vi "FFT_polynomial_bkg.vi"(8 "Y-column names":string[](array[string])=["col0"], 10 "column extension":string[](array[string])=["summer school 206.006.text"], 11 "Graph array":cluster{"output":dbl[], "output":dbl[]}[](array[cluster])=[{"output"=array[1000 elements], "output"=array[1000 elements]}]) -> ()   [LabVIEW 2025]
uses:
  <vilib>/Analysis/1siggen.llb/Ramp Pattern by Samples.vi
  <vilib>/Analysis/4window.llb/Welch Window (DBL).vi
  <vilib>/Analysis/4window.llb/Triangle Window (DBL).vi
  <vilib>/Analysis/4window.llb/Modified Bartlett-Hanning Window (DBL).vi
  <vilib>/Analysis/4window.llb/Hanning Window (DBL).vi
  <vilib>/Analysis/4window.llb/Hamming Window (DBL).vi
  <vilib>/Analysis/4window.llb/Blackman Window (DBL).vi
  <vilib>/Analysis/2dsp.llb/Power Spectrum (DBL).vi
  <vilib>/Analysis/4window.llb/AllCosWindow (DBL).vi
  <vilib>/Analysis/NI_AALPro.lvlib
  <vilib>/Analysis/NI_AALBase.lvlib
  <vilib>/gmath/NI_Gmath.lvlib
panel:
  in  "length":i32=1000
  in  "index":i32
  in  "bkg removal":enum16{"divide", "subtract"}(ring)
  in  "data":enum16{"spectrum", "1/B plot"}(ring)
  out "1/(x-scale range)":dbl
  in  "show accumulative spectrums":bool
  out "x-array":dbl[](array[numeric])
  in  "export":T1(ring)=enum."write to clipboard"
  in  "data offset":dbl format="%.2e"
  in  "use 1/B for fit":bool
  in  "Bbkg final":dbl=22.0 format="%.2f"
  in  "Bbkg init":dbl=13.0 format="%.2f"
  in  "bkg removal method":enum16{"polynomial", "Cheby poly"}(ring)
  out "raw data/bkg":T2(graph)
  out "FFT spectrum":cluster{"all rows":dbl[], "all rows":dbl[]}[](graph)
  in  "interpol. method":i32(ring)=2 items=["nearest", "linear", "spline", "cubic Hermite", "Lagrange"]
  in  "window":T3(ring)=enum."Hanning"
  in  "stop":bool
  in  "use variables":bool
  in  "Interpolation #":i32=5000
  in  "export results":bool
  out "Field, Freq., Amp":string="0.000E+0\t2.237E+2\r\n"
  out "FFT freq":cluster{"array type (2D Dbl)":dbl[], dbl[]}(graph)={"array type (2D Dbl)"=[0.0], [223.74319564521292]}
  out "FFT amp":cluster{"array type (2D Dbl)":dbl[], dbl[]}(graph)={"array type (2D Dbl)"=[0.0], [8.187351253588833e-05]}
  out "Windowed Signal":cluster{"all rows":dbl[], "all rows":dbl[]}[](graph)
  in  "bkg poly. order":i32=2
  in  "B final":dbl=22.0 format="%.2f"
  in  "B init":dbl=13.0 format="%.2f"
  out "1/B plot after bkg removed":cluster{"all rows":dbl[], "all rows":dbl[]}[](graph)
  in  "variable":string="4.2\n3.5\n3"
  # "Turn on the Show Context Help option ON for\na brief explanation of the controls and graphs."
  # "1. Background removal is done by fitting (normal or Chebyshev polynomial) \n   i) Fitting is done for the range given by 'Bbkg init' and 'Bbkg final'.\n   ii) Background curve is extended to the range give by 'B init' and 'B final'.\n\n2. FFT is done in the range given by 'B init' and 'B final'."
  # "The position and amplitude of the peak will appear on the right two panels. \nOne can zoom in or out to focus on specific peaks."
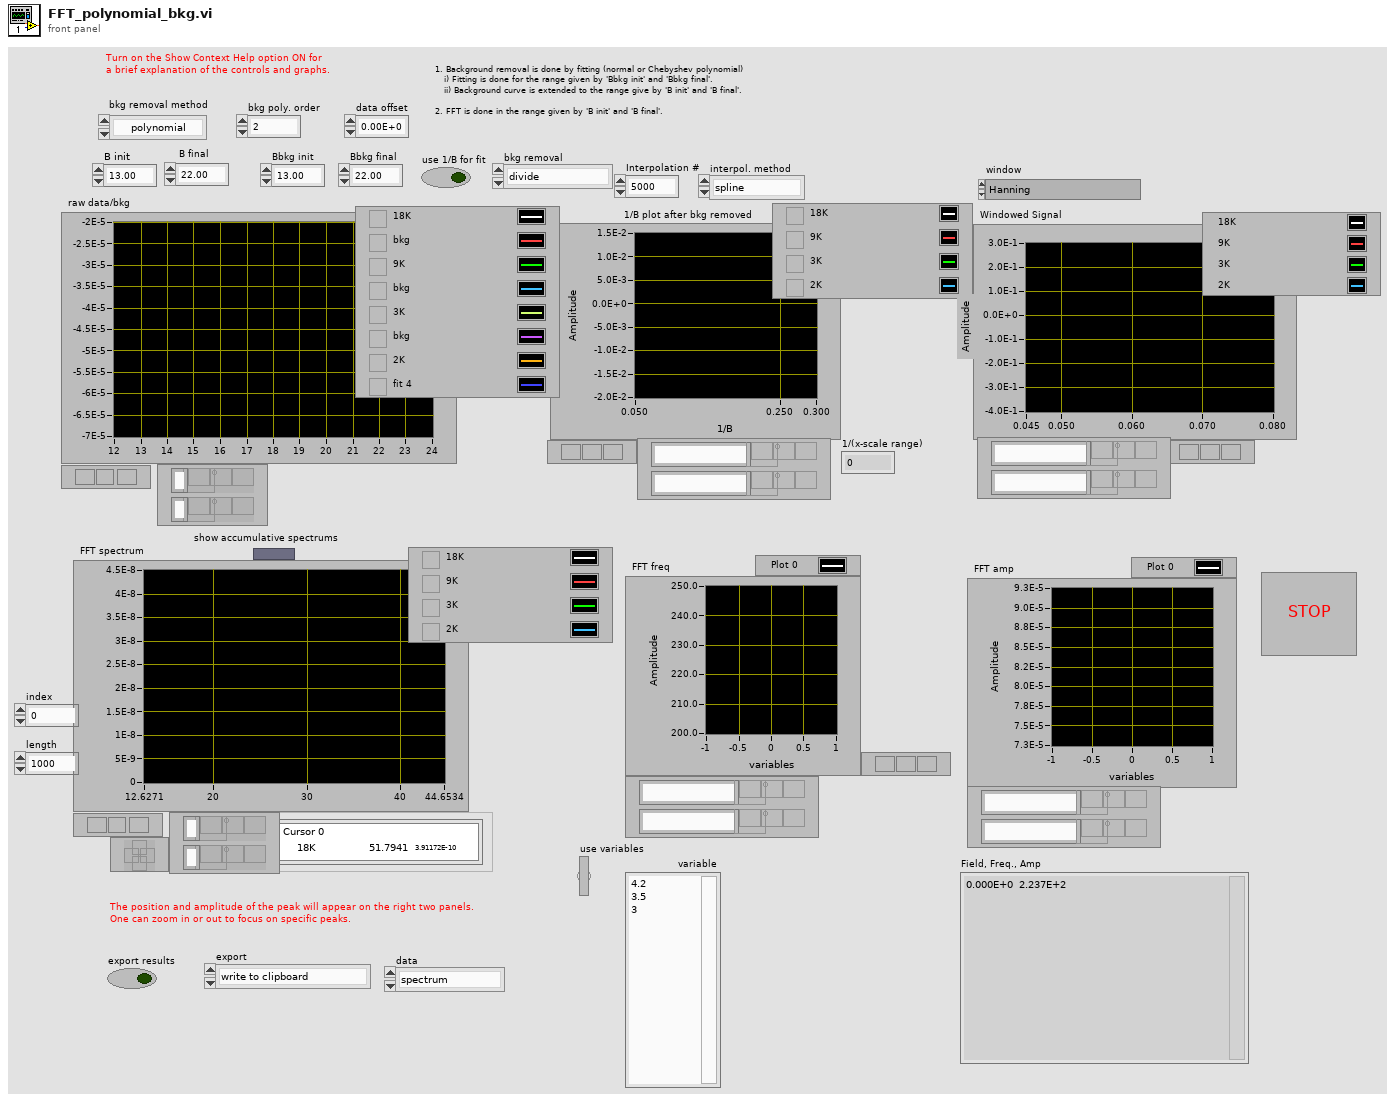
[diagram p1: front panel]
types:
  T1 = enum16{"Save as Ascill file", "write to clipboard", "write to Igor ITX file"}
  T2 = cluster{"Ramp Pattern":dbl[], "Power Spectrum":dbl[]}[]
  T3 = enum16{"none", "Welch", "Triangular", "Bartlett", "Hanning", "Hamming", "Blackmann"}
  T4 = enum16{"Save as Ascill file", "write to clipboard", "do not export"}
  T5 = cluster{"extended B":dbl[], "extended data":dbl[]}
  T6 = cluster{"xi used":dbl[], "Zero Padded Array":dbl[]}
  T7 = cluster{"xi used":dbl[], "Zero Padded Array":dbl[]}[]
  T8 = cluster{"extended B":dbl[], "extended data":dbl[]}[]
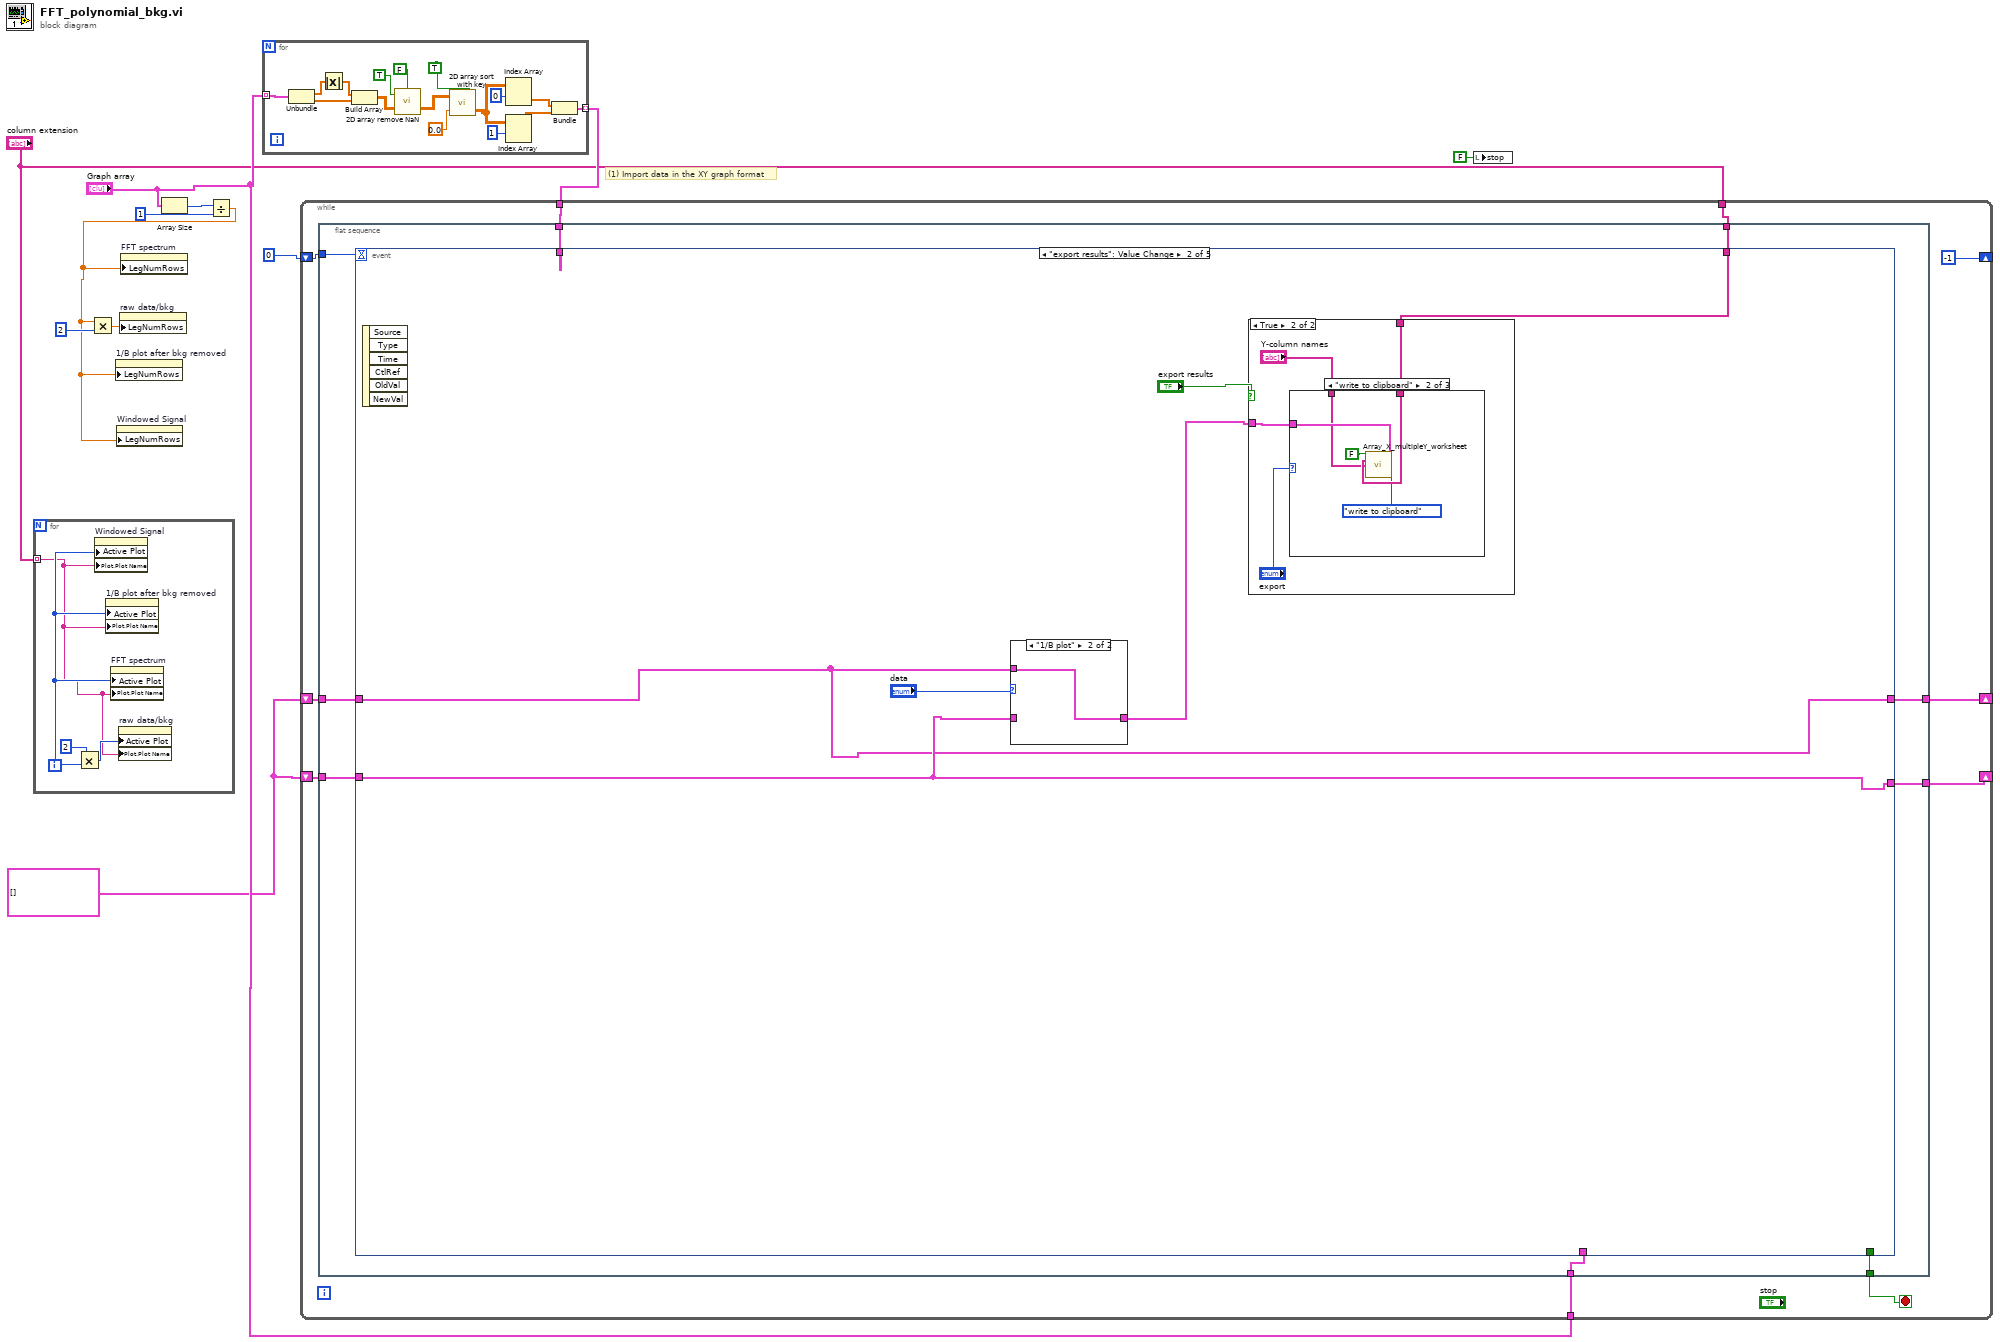
[diagram p0: block diagram]
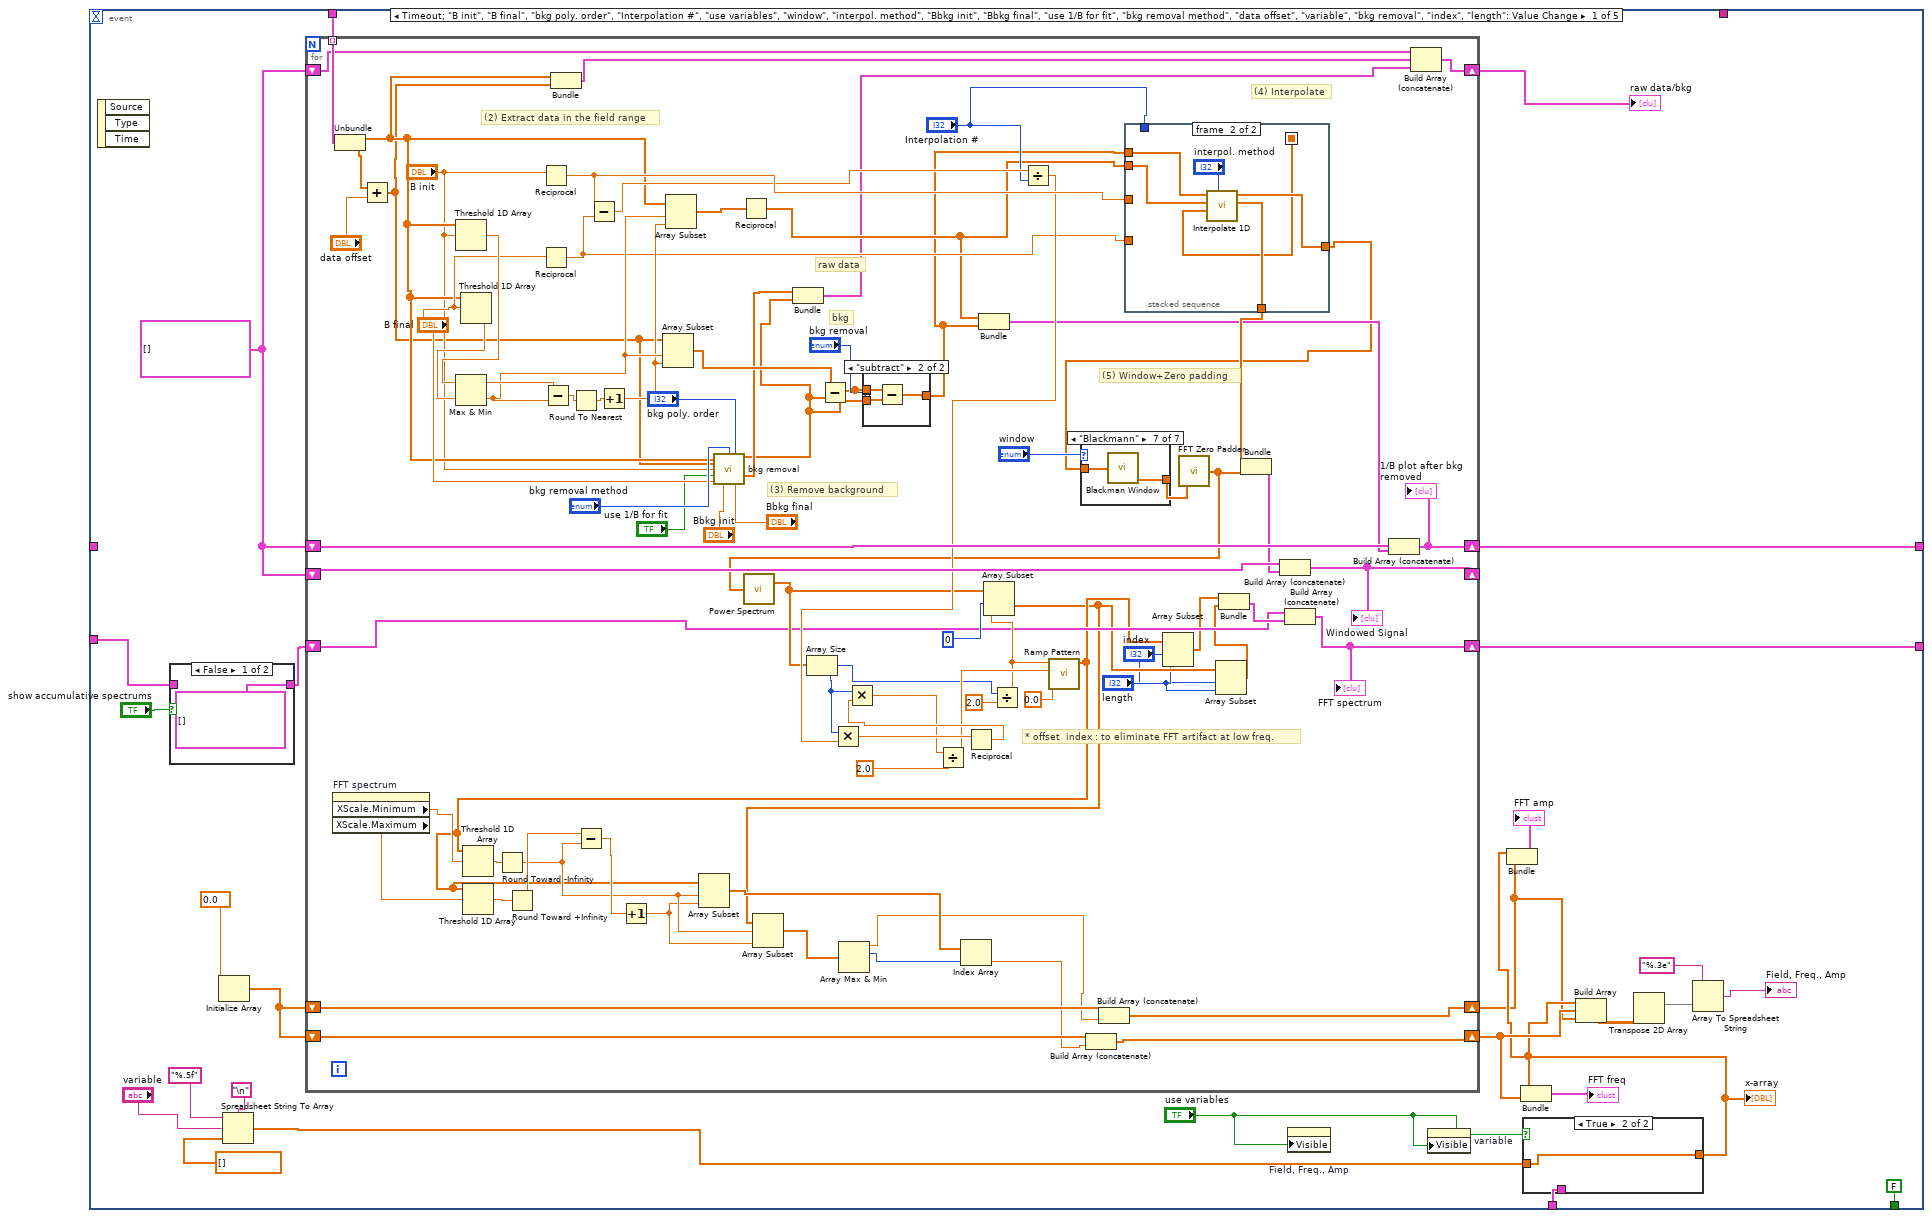
[diagram p2: hidden frame]
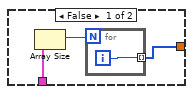
[diagram p4: hidden frame]
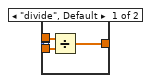
[diagram p5: hidden frame]
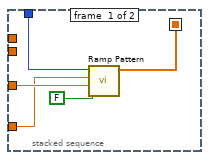
[diagram p6: hidden frame]
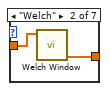
[diagram p8: hidden frame]
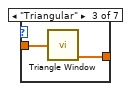
[diagram p9: hidden frame]
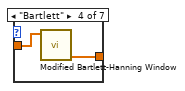
[diagram p10: hidden frame]
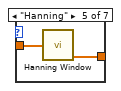
[diagram p11: hidden frame]
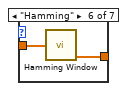
[diagram p12: hidden frame]
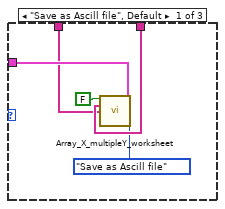
[diagram p15: hidden frame]
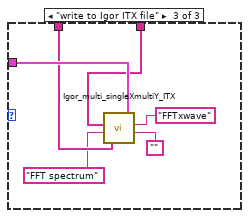
[diagram p16: hidden frame]
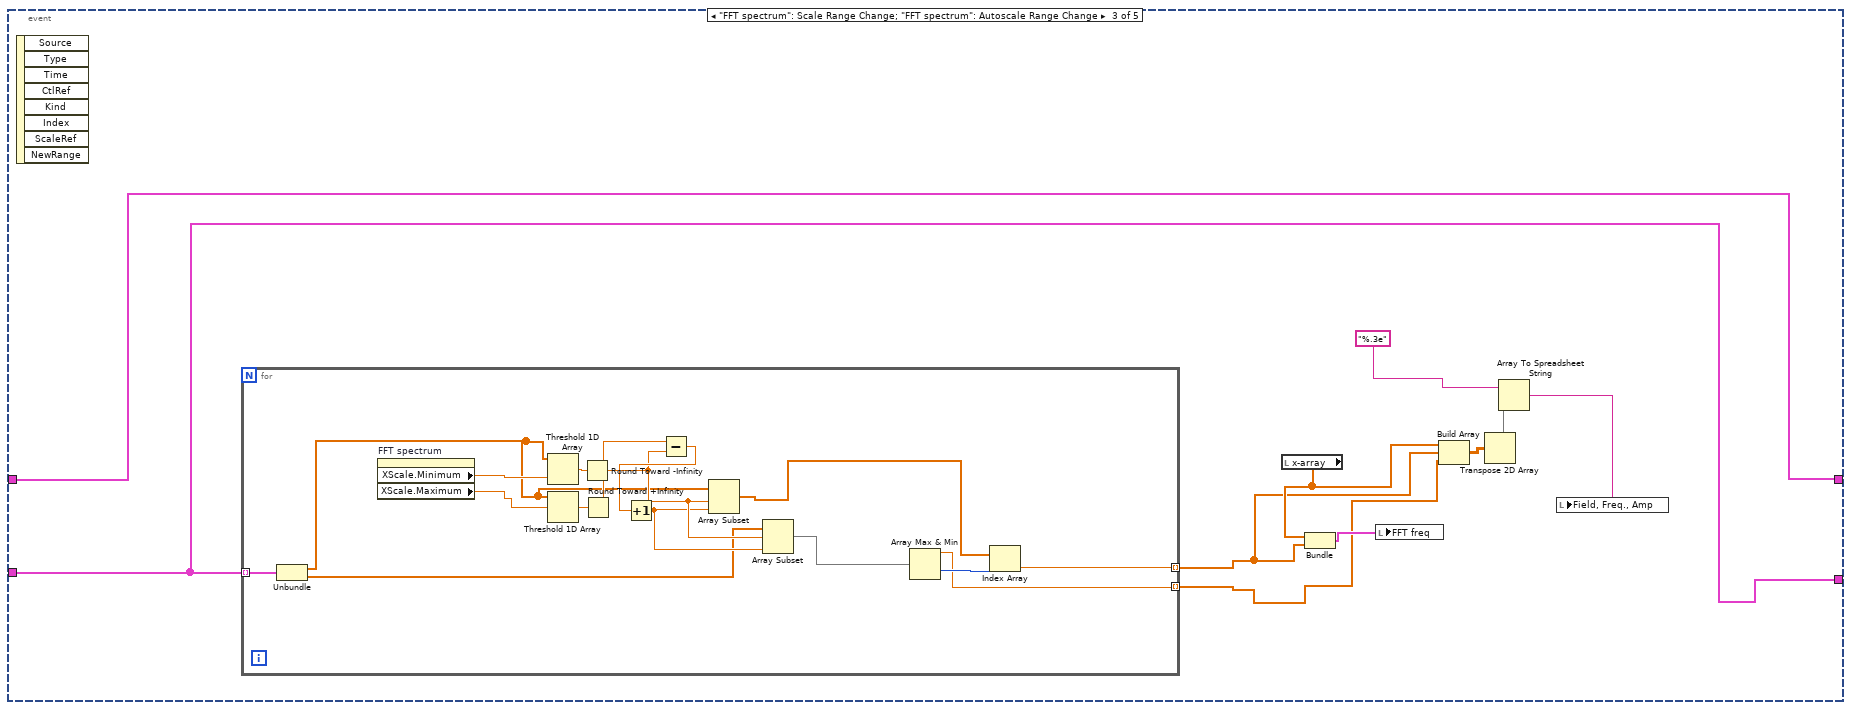
[diagram p17: hidden frame]
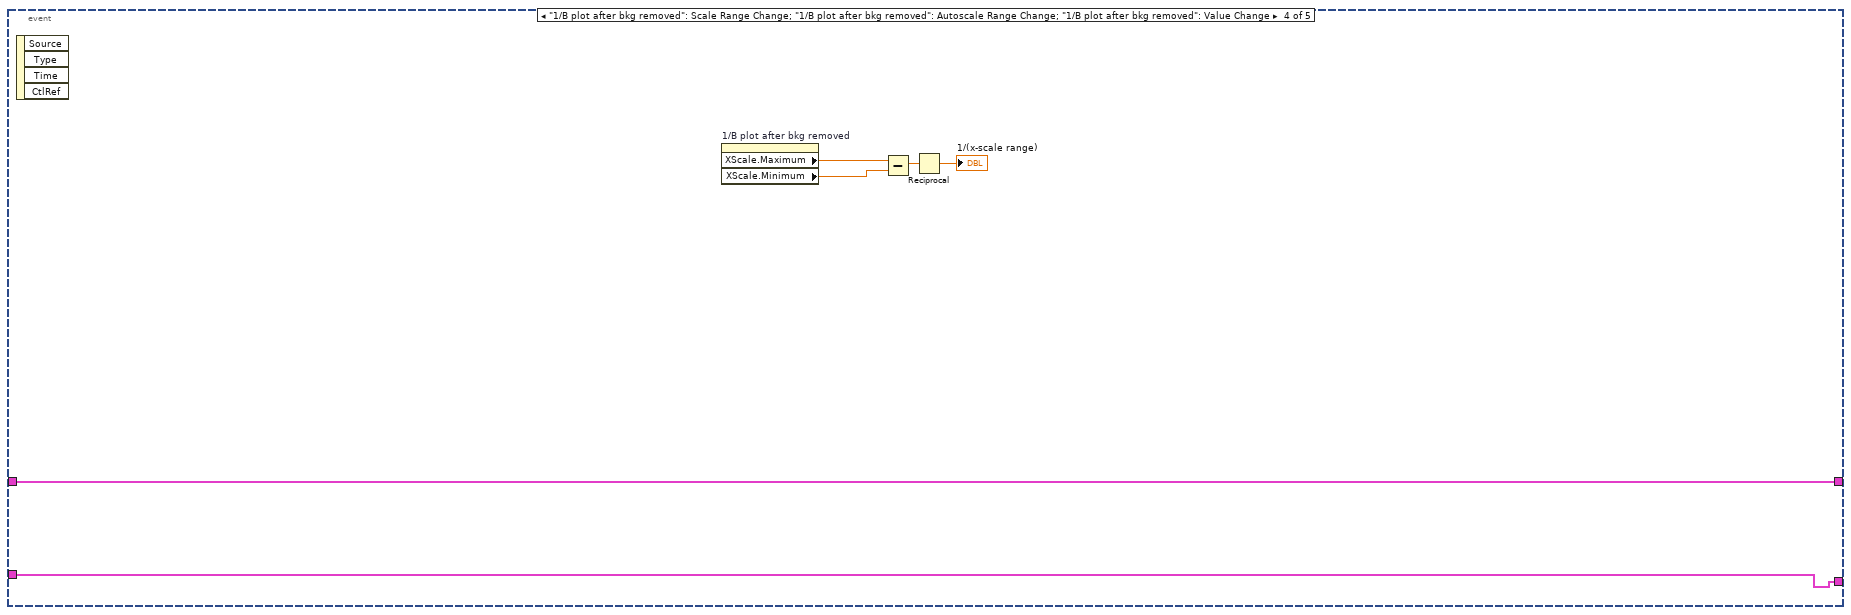
[diagram p18: hidden frame]
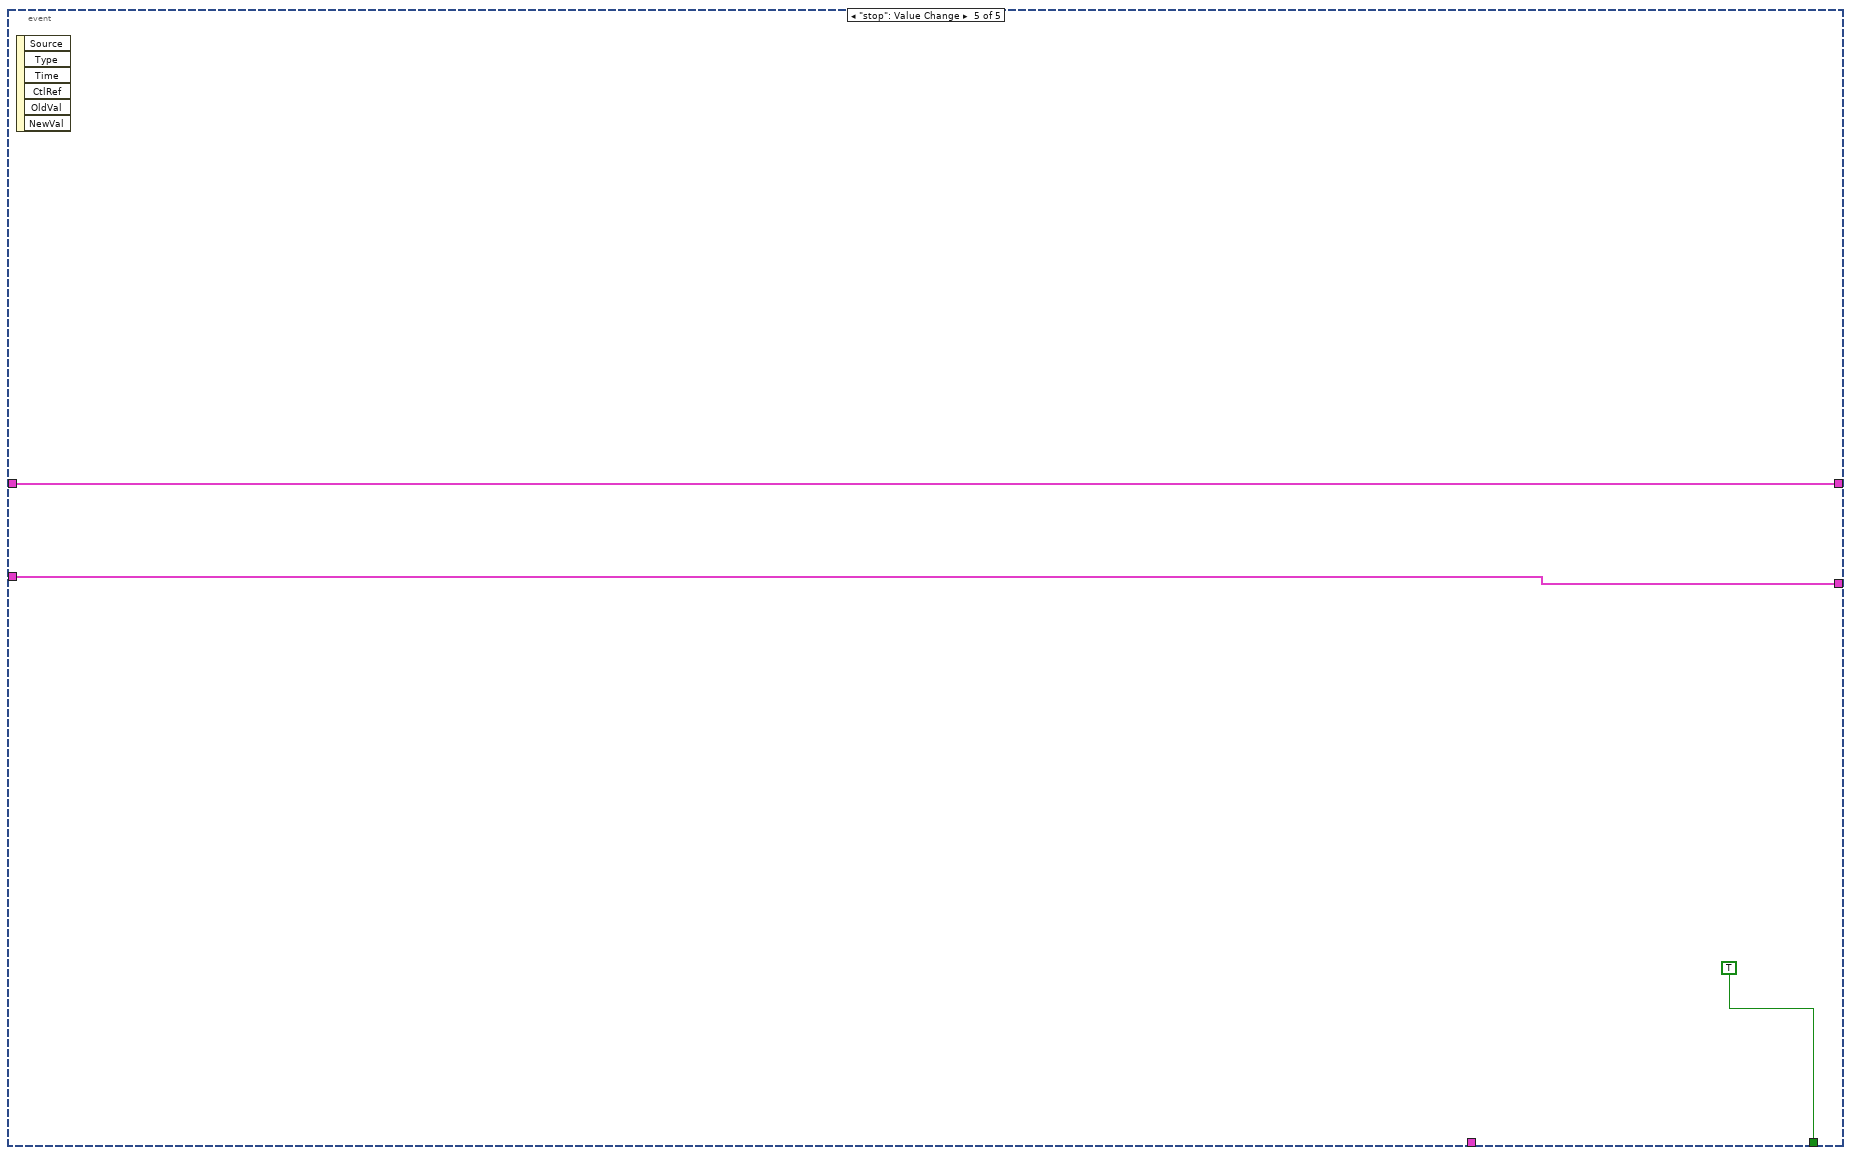
[diagram p19: hidden frame]
diagram:
  w4 = cluster{"all rows":sgl[], "all rows":sgl[]}[] []
  # "(1) Import data in the XY graph format"
  n1 = for {
    tunnel: "column extension" -> [w12] mode=indexing
    i -> [w15]
    n2 = Multiply(x=2, y=w15) -> (x*y=w13:i32)
    n3 = property on="Windowed Signal" class="XYGraph (strict)"("Active Plot"=w15, "Plot.Plot Name"=w12) -> ()  [unwired: 2 in, 2 out]
    n4 = property on="1/B plot after bkg removed" class="XYGraph (strict)"("Active Plot"=w15, "Plot.Plot Name"=w12) -> ()  [unwired: 2 in, 2 out]
    n5 = property on="FFT spectrum" class="XYGraph (strict)"("Active Plot"=w15, "Plot.Plot Name"=w12) -> ()  [unwired: 2 in, 2 out]
    n6 = property on="raw data/bkg" class="XYGraph (strict)"("Active Plot"=w13, "Plot.Plot Name"=w12) -> ()  [unwired: 2 in, 2 out]
  }
  n7 = Array Size(array="Graph array") -> (size(s)=w3:i32)
  n8 = Divide(x=w3, y=1) -> (x/y=w1:dbl)
  n9 = Multiply(x=w1, y=2) -> (x*y=w7:dbl)
  n10 = property on="1/B plot after bkg removed" class="XYGraph (strict)"("LegNumRows"=w1) -> ()  [unwired: 2 in, 2 out]
  n11 = property on="Windowed Signal" class="XYGraph (strict)"("LegNumRows"=w1) -> ()  [unwired: 2 in, 2 out]
  n12 = property on="raw data/bkg" class="XYGraph (strict)"("LegNumRows"=w7) -> ()  [unwired: 2 in, 2 out]
  n13 = property on="FFT spectrum" class="XYGraph (strict)"("LegNumRows"=w1) -> ()  [unwired: 2 in, 2 out]
  n14 = for {
    tunnel: "Graph array" -> [w31] mode=indexing
    tunnel: [w21] -> w10 mode=indexing
    n15 = Unbundle(w31) -> ("output"=w29:dbl[], "output"=w28:dbl[])
    n16 = Absolute Value(x=w29) -> (abs(x)=w20:dbl[])
    n17 = Build Array(w20, w28) -> (w19:dbl[][])
    n18 = call "2D array remove NaN.vi"("Data array"=FALSE, "2D array IN"=w19, "delete Nan"=TRUE) -> ("2D array cleaned"=w18:dbl[][])
    n19 = call "2D array sort with key.vi"("ascending"=TRUE, "key row"=0.0, "input"=w18) -> ("output"=w26:dbl[][])
    n20 = Index Array(array=w26, index (row)=0) -> (element=w23:dbl[])  [unwired: 1 in]
    n21 = Index Array(array=w26, index (row)=1) -> (element=w22:dbl[])  [unwired: 1 in]
    n22 = Bundle("output"=w23, "output"=w22) -> (w21:cluster{"output":dbl[], "output":dbl[]})  [unwired: 1 in]
  }
  n23 = while {
    tunnel: w10 -> [w41]
    tunnel: "Graph array" -> [w40]
    shift-right: [-1] -> _
    shift-left: 0 -> [w38]
    tunnel: "column extension" -> [w36]
    shift-right: [w35] -> _
    shift-left: w4 -> [w34]
    shift-right: [w33] -> _
    shift-left: w4 -> [w32]
    stop <- w39 stop-if-true
    n24 = flat-sequence {
      tunnel: w41 -> [w50]
      tunnel: w40 -> [w49]
      tunnel: [w48] -> w39
      tunnel: w38 -> [w47]
      tunnel: w36 -> [w46]
      tunnel: [w45] -> w35
      tunnel: w34 -> [w44]
      tunnel: [w43] -> w33
      tunnel: w32 -> [w42]
      frame #0 {
        n25 = event shown="[1] \"export results\": Value Change" {
          selector: _ -> [_ _ _ _ _]
          dyn-events: _ -> [_ _ _ _ _]
          timeout: w47 -> [_ _ _ _ _]
          tunnel: w50 -> [w65 _ _ _ _]
          tunnel: w49 -> [w62 _ _ _ _]
          tunnel: [FALSE ("stop (press twice)") _ _ _ TRUE ("stop (press twice)")] -> w48
          tunnel: w46 -> [w57 w204 _ _ _]
          tunnel: [w57 _ _ _ _] -> _
          tunnel: [w56 w202 w230 w255 w261] -> w45
          tunnel: w44 -> [w54 w202 w230 w255 w261]
          tunnel: [w52 w200 w229 w254 w260] -> w43
          tunnel: w42 -> [_ w200 w229 w254 w260]
          event Timeout; "B init", "B final", "bkg poly. order", "Interpolation #", "use variables", "window", "interpol. method", "Bbkg init", "Bbkg final", "use 1/B for fit", "bkg removal method", "data offset", "variable", "bkg removal", "index", "length": Value Change {
            w58 = cluster{"all rows":sgl[], "all rows":sgl[]}[] []
            n26 = event-data() -> ()  [unwired: 1 in, 3 out]
            n27 = case shown="False" "show accumulative spectrums" {
              tunnel: w54 -> [_ w80]
              tunnel: [cluster{"all rows":sgl[], "all rows":sgl[]}[] [] w80] -> w53
              frame False {
              }
              frame True {
              }
            }
            n28 = Initialize Array(0.0 ("element")) -> (w77:dbl[])  [unwired: 1 in]
            n29 = Spreadsheet String To Array(delimiter (Tab)="\n", format string="%.5f", spreadsheet string="variable", array type (2D Dbl)=dbl[] []) -> (array=w63:dbl[])
            n30 = for {
              shift-right: [w152] -> w52
              shift-left: w58 -> [w168]
              shift-right: [w151] -> _
              shift-left: w58 -> [w163]
              shift-right: [w132] -> w56
              shift-left: w53 -> [w96]
              shift-right: [w150] -> w51
              shift-left: w77 -> [w154]
              shift-right: [w149] -> w71
              shift-left: w77 -> [w153]
              tunnel: w65 -> [w147] mode=indexing
              shift-right: [w131] -> w59
              shift-left: w58 -> [w130]
              # "(5) Window+Zero padding"
              # "(4) Interpolate"
              # "(3) Remove background"
              # "(2) Extract data in the field range"
              # "bkg"
              # "raw data"
              # "* offset  index : to eliminate FFT artifact at low freq."
              n31 = property on="FFT spectrum" class="XYGraph (strict)"() -> ("XScale.Minimum"=w100:dbl, "XScale.Maximum"=w99:dbl)  [unwired: 2 in, 2 out]
              n32 = Unbundle(w147) -> ("output"=w120:dbl[], "output"=w113:dbl[])
              n33 = Add(x=w113, y="data offset") -> (x+y=w111:dbl[])
              n34 = Threshold 1D Array(2:"B init", 3:w120) -> (0:w167:dbl)  [unwired: 1 in]
              n35 = Threshold 1D Array(2:"B final", 3:w120) -> (0:w166:dbl)  [unwired: 1 in]
              n36 = Max & Min(x=w167, y=w166) -> (max(x,y)=w165:dbl, min(x,y)=w161:dbl)
              n37 = Reciprocal(x="B init") -> (1/x=w160:dbl)
              n38 = Reciprocal(x="B final") -> (1/x=w143:dbl)
              n39 = Subtract(x=w165, y=w161) -> (x-y=w164:dbl)
              n40 = Bundle("output"=w120, w111) -> (w119:cluster{"output":dbl[], dbl[]})  [unwired: 1 in]
              n41 = Round To Nearest(number=w164) -> (nearest integer value=w169:dbl)
              n42 = Subtract(x=w160, y=w143) -> (x-y=w158:dbl)
              n43 = Increment(x=w169) -> (x+1=w159:dbl)
              n44 = Array Subset(array=w111, index=w161, length=w159) -> (w129:dbl[])
              n45 = Array Subset(array=w120, index=w161, length=w159) -> (w118:dbl[])
              n46 = call "bkg removal.vi"("Bfield"=w120, "bkg removal method"="bkg removal method", "poly. order"="bkg poly. order", "Data"=w111, "B initial"="B init", "inverse"="use 1/B for fit", "B final"="B final", "Bbkg initial"="Bbkg init", "Bbkg final"="Bbkg final") -> ("extended data"=w94:dbl[], "extended B"=w116:dbl[])  [unwired: 4 in, 1 out]
              n47 = Reciprocal(x=w118) -> (1/x=w126:dbl[])
              n48 = Bundle("extended B"=w116, "extended data"=w94) -> (w115:T5)  [unwired: 1 in]
              n49 = Subtract(x=w129, y=w94) -> (x-y=w92:dbl[])
              n50 = case shown="\"subtract\"" "bkg removal" {
                tunnel: w92 -> [w172 _]
                tunnel: w94 -> [w171 w174]
                tunnel: [w170 w173] -> w93
                tunnel: w92 -> [_ w175]
                frame "divide", Default {
                  n51 = Divide(x=w172, y=w171) -> (x/y=w170:dbl[])
                }
                frame "subtract" {
                  n52 = Subtract(x=w175, y=w174) -> (x-y=w173:dbl[])
                }
              }
              n53 = Bundle(w126, w93) -> (w128:cluster{dbl[], dbl[]})  [unwired: 1 in]
              n54 = Divide(x=w158, y="Interpolation #") -> (x/y=w156:dbl)
              n55 = stacked-sequence {
                seq-local: [w176 _] -> [_ w181]
                tunnel: w93 -> [_ w186]
                tunnel: w126 -> [_ w185]
                tunnel: [_ w184] -> w144
                tunnel: [_ w183] -> w127
                tunnel: "Interpolation #" -> [w180 _]
                tunnel: w160 -> [w179 _]
                tunnel: w143 -> [w178 _]
                frame #0 {
                  n56 = call-poly <vilib>:"Ramp Pattern.vi"("exclude end?"=FALSE, "start"=w179, "end"=w178, "samples"=w180) -> ("Ramp Pattern"=w176:dbl[])  [unwired: 6 in, 1 out]
                }
                frame #1 {
                  n57 = call <vilib>:"Interpolate 1D.vi"("method"="interpol. method", "xi"=w181, "X"=w185, "Y"=w186) -> ("xi used"=w184:dbl[], "yi"=w183:dbl[])  [unwired: 5 in, 1 out]
                }
              }
              n58 = case shown="\"Blackmann\"" "window" {
                tunnel: [w187 w189 w191 w193 w195 w197 w199] -> w157
                tunnel: w127 -> [w187 w188 w190 w192 w194 w196 w198]
                frame "none" {
                }
                frame "Welch" {
                  n59 = call-poly <vilib>:"Welch Window.vi"("X"=w188) -> ("Windowed X"=w189:dbl[])  [unwired: 9 in, 1 out]
                }
                frame "Triangular" {
                  n60 = call-poly <vilib>:"Triangle Window.vi"("X"=w190) -> ("Windowed X"=w191:dbl[])  [unwired: 1 out]
                }
                frame "Bartlett" {
                  n61 = call-poly <vilib>:"Modified Bartlett-Hanning Window.vi"("X"=w192) -> ("Windowed X"=w193:dbl[])  [unwired: 9 in, 1 out]
                }
                frame "Hanning" {
                  n62 = call-poly <vilib>:"Hanning Window.vi"("X"=w194) -> ("Windowed X"=w195:dbl[])  [unwired: 1 out]
                }
                frame "Hamming" {
                  n63 = call-poly <vilib>:"Hamming Window.vi"("X"=w196) -> ("Windowed X"=w197:dbl[])  [unwired: 1 out]
                }
                frame "Blackmann" {
                  n64 = call-poly <vilib>:"Blackman Window.vi"("X"=w198) -> ("Windowed X"=w199:dbl[])  [unwired: 1 out]
                }
              }
              n65 = call "FFT Zero Padder.vi"("Input Array"=w157) -> ("Zero Padded Array"=w155:dbl[])  [unwired: 1 in]
              n66 = call-poly <vilib>:"Power Spectrum.vi"("X"=w155) -> ("Power Spectrum"=w134:dbl[])  [unwired: 1 out]
              n67 = Array Size(array=w134) -> (size(s)=w135:i32)
              n68 = Multiply(x=w135, y=w156) -> (x*y=w148:dbl)
              n69 = Reciprocal(x=w148) -> (1/x=w142:dbl)
              n70 = Multiply(x=w135, y=w142) -> (x*y=w140:dbl)
              n71 = Divide(x=w140, y=2.0) -> (x/y=w139:dbl)
              n72 = Divide(x=w135, y=2.0) -> (x/y=w133:dbl)
              n73 = Array Subset(array=w134, index=0, length=w133) -> (w90:dbl[])
              n74 = call-poly <vilib>:"Ramp Pattern.vi"("start"=0.0, "end"=w139, "samples"=w133) -> ("Ramp Pattern"=w91:dbl[])  [unwired: 7 in, 1 out]
              n75 = Threshold 1D Array(2:w100, 3:w91) -> (0:w108:dbl)  [unwired: 1 in]
              n76 = Threshold 1D Array(2:w99, 3:w91) -> (0:w109:dbl)  [unwired: 1 in]
              n77 = Round Toward -Infinity(1:w108) -> (0:w105:dbl)
              n78 = Round Toward +Infinity(x=w109) -> (ceil(x): smallest int >= x=w107:dbl)
              n79 = Subtract(x=w107, y=w105) -> (x-y=w106:dbl)
              n80 = Increment(x=w106) -> (x+1=w104:dbl)
              n81 = Array Subset(array=w91, index=w105, length=w104) -> (w102:dbl[])
              n82 = Array Subset(array=w90, index=w105, length=w104) -> (w103:dbl[])
              n83 = Array Max & Min(array=w103) -> (max value=w98:dbl, max index (indices)=w101:i32)  [unwired: 2 out]
              n84 = Index Array(array=w102, index=w101) -> (element=w97:dbl)
              n85 = Build Array (concatenate)(w153, w97) -> (w149:dbl[])
              n86 = Build Array (concatenate)(w154, w98) -> (w150:dbl[])
              n87 = Array Subset(array=w91, index="index", length="length") -> (w87:dbl[])
              n88 = Array Subset(array=w90, index="index", length="length") -> (w86:dbl[])
              n89 = Bundle(w87, w86) -> (w138:cluster{dbl[], dbl[]})  [unwired: 1 in]
              n90 = Bundle("xi used"=w144, "Zero Padded Array"=w155) -> (w162:T6)  [unwired: 1 in]
              n91 = Build Array (concatenate)(w163, w162) -> (w151:T7)
              "Windowed Signal" <- w151
              n92 = Build Array (concatenate)(w96, w138) -> (w132:cluster{"all rows":dbl[], "all rows":dbl[]}[])
              "FFT spectrum" <- w132
              n93 = Build Array (concatenate)(w168, w128) -> (w152:cluster{"all rows":dbl[], "all rows":dbl[]}[])
              "1/B plot after bkg removed" <- w152
              n94 = Build Array (concatenate)(w130, w119, w115) -> (w131:T8)
            }
            "raw data/bkg" <- w59
            n95 = property on="Field, Freq., Amp" class="Str"("Visible"="use variables") -> ()  [unwired: 2 in, 2 out]
            n96 = property on="variable" class="Str"("Visible"="use variables") -> ()  [unwired: 2 in, 2 out]
            n97 = case shown="True" "use variables" {
              tunnel: w63 -> [_ w85]
              tunnel: [w82 w85] -> w64
              tunnel: w62 -> [w81 _]
              frame False {
                n98 = Array Size(array=w81) -> (size(s)=w83:i32)
                n99 = for {
                  N: w83 -> [_]
                  tunnel: [w84] -> w82 mode=indexing
                  i -> [w84]
                }
              }
              frame True {
              }
            }
            "x-array" <- w64
            n100 = Bundle("array type (2D Dbl)"=w64, w51) -> (→"FFT amp":cluster{"array type (2D Dbl)":dbl[], dbl[]})  [unwired: 1 in]
            n101 = Bundle("array type (2D Dbl)"=w64, w71) -> (→"FFT freq":cluster{"array type (2D Dbl)":dbl[], dbl[]})  [unwired: 1 in]
            n102 = Build Array(w64, w71, w51) -> (w76:dbl[][])
            n103 = Transpose 2D Array(2D array=w76) -> (transposed array=w75:dbl[][])
            n104 = Array To Spreadsheet String(array=w75, 3:"%.3e" ("format string")) -> (spreadsheet string=→"Field, Freq., Amp":string)  [unwired: 1 in]
          }
          event "export results": Value Change {
            n105 = event-data() -> ()  [unwired: 1 in, 6 out]
            n106 = case shown="\"1/B plot\"" "data" {
              tunnel: w202 -> [w206 _]
              tunnel: [w206 w207] -> w201
              tunnel: w200 -> [_ w207]
              frame "spectrum", Default {
              }
              frame "1/B plot" {
              }
            }
            n107 = case shown="True" "export results" {
              tunnel: w201 -> [_ w210]
              tunnel: w204 -> [_ w208]
              frame False {
              }
              frame True {
                n108 = case shown="\"write to clipboard\"" "export" {
                  tunnel: w210 -> [w216 w221 w227]
                  tunnel: w208 -> [w214 w219 w226]
                  tunnel: "Y-column names" -> [w213 w218 w225]
                  frame "Save as Ascill file", Default {
                    n109 = call "Array_X_multipleY_worksheet.vi"("Sort?"=FALSE, "graph file"=w216, "column extension"=w214, "Y-column names"=w213, "export"=T4."Save as Ascill file") -> ()  [unwired: 9 in, 2 out]
                  }
                  frame "write to clipboard" {
                    n110 = call "Array_X_multipleY_worksheet.vi"("Sort?"=FALSE, "graph file"=w221, "column extension"=w219, "Y-column names"=w218, "export"=T4."write to clipboard") -> ()  [unwired: 9 in, 2 out]
                  }
                  frame "write to Igor ITX file" {
                    n111 = call "Igor_multi_singleXmultiY_ITX.vi"("message"="", "x-column name"="FFTxwave", "graph file"=w227, "Y-column names"=w225, "window name"="FFT spectrum", "column extension"=w226) -> ()  [unwired: 1 in, 1 out]
                  }
                }
              }
            }
          }
          event "FFT spectrum": Scale Range Change; "FFT spectrum": Autoscale Range Change {
            n112 = event-data() -> ()  [unwired: 1 in, 8 out]
            n113 = for {
              tunnel: w230 -> [w242] mode=indexing
              tunnel: [w239] -> w233 mode=indexing
              tunnel: [w238] -> w228 mode=indexing
              n114 = Unbundle(w242) -> ("all rows"=w241:dbl[], "all rows"=w240:dbl[])
              n115 = property on="FFT spectrum" class="XYGraph (strict)"() -> ("XScale.Minimum"=w253:dbl, "XScale.Maximum"=w252:dbl)  [unwired: 2 in, 2 out]
              n116 = Threshold 1D Array(2:w253, 3:w241) -> (0:w250:dbl)  [unwired: 1 in]
              n117 = Threshold 1D Array(2:w252, 3:w241) -> (0:w251:dbl)  [unwired: 1 in]
              n118 = Round Toward -Infinity(1:w250) -> (0:w247:dbl)
              n119 = Round Toward +Infinity(x=w251) -> (ceil(x): smallest int >= x=w249:dbl)
              n120 = Subtract(x=w249, y=w247) -> (x-y=w248:dbl)
              n121 = Increment(x=w248) -> (x+1=w246:dbl)
              n122 = Array Subset(array=w241, index=w247, length=w246) -> (w244:dbl[])
              n123 = Array Subset(array=w240, index=w247, length=w246) -> (w245:dbl[])
              n124 = Array Max & Min(array=w245) -> (max value=w238:dbl, max index (indices)=w243:i32)  [unwired: 2 out]
              n125 = Index Array(array=w244, index=w243) -> (element=w239:dbl)
            }
            n126 = local read "x-array"() -> (w234:dbl[])
            n127 = Bundle("x-array"=w234, w233) -> (w231:cluster{"x-array":dbl[], dbl[]})  [unwired: 1 in]
            n128 = local write "FFT freq"(w231) -> ()
            n129 = Build Array(w234, w233, w228) -> (w236:dbl[][])
            n130 = Transpose 2D Array(2D array=w236) -> (transposed array=w237:dbl[][])
            n131 = Array To Spreadsheet String(array=w237, 3:"%.3e" ("format string")) -> (spreadsheet string=w232:string)  [unwired: 1 in]
            n132 = local write "Field, Freq., Amp"(w232) -> ()
          }
          event "1/B plot after bkg removed": Scale Range Change; "1/B plot after bkg removed": Autoscale Range Change; "1/B plot after bkg removed": Value Change {
            n133 = event-data() -> ()  [unwired: 1 in, 4 out]
            n134 = property on="1/B plot after bkg removed" class="XYGraph (strict)"() -> ("XScale.Maximum"=w259:dbl, "XScale.Minimum"=w258:dbl)  [unwired: 2 in, 2 out]
            n135 = Subtract(x=w259, y=w258) -> (x-y=w257:dbl)
            n136 = Reciprocal(x=w257) -> (1/x=→"1/(x-scale range)":dbl)
          }
          event "stop": Value Change {
            n137 = event-data() -> ()  [unwired: 1 in, 6 out]
          }
        }
      }
    }
  }
  n138 = local write "stop"(FALSE ("stop")) -> ()
